vi "4024_Module_configure.vi"() -> ()   [LabVIEW 2020]
panel:
  in  "Output Range":u16(ring)=2 items=["30   0 to 20mA", "31   4 to 20mA", "32   0 to 10V"]
  in  "Ch Number":i8
  in  "Port Name":string="COM10"
  out "Reply":string
  out "ConfigStringSent":string
  in  "Address":u8
  # "This is a per channel configuration \nto be done after you have run \n4024_Module_INIT_configure.vi \n\nDon't run this vi when the ADAM 4024 is in the INIT mode"
  # "Happy reply starts \"!\"\nUnhappy reply starts \"?\""
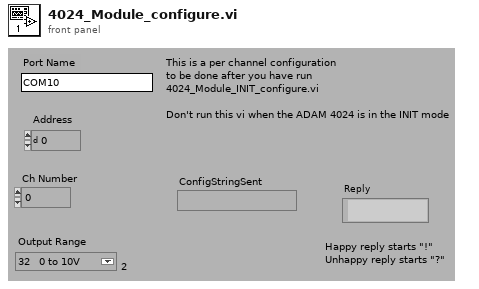
[diagram p1: front panel]
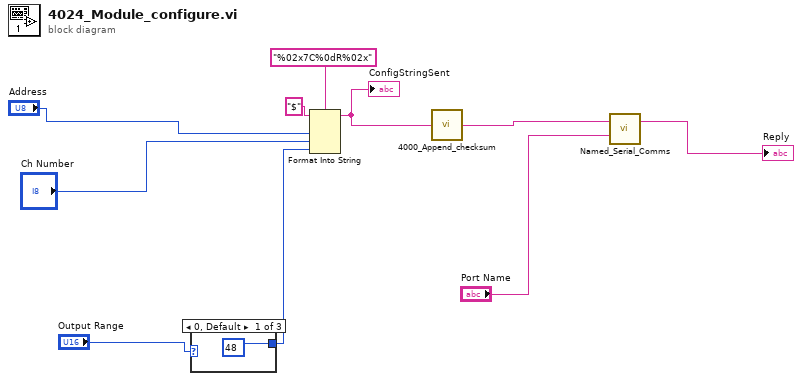
[diagram p0: block diagram]
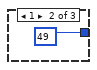
[diagram p2: hidden frame]
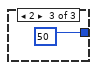
[diagram p3: hidden frame]
diagram:
  n1 = case shown="0, Default" "Output Range" {
    tunnel: [48 49 50] -> w1
    frame 0, Default {
    }
    frame 1 {
    }
    frame 2 {
    }
  }
  n2 = Format Into String(format string="%02x7C%0dR%02x", initial string="$", "Address", "Ch Number", w1) -> (resulting string=w8:string)  [unwired: 1 in, 1 out]
  "ConfigStringSent" <- w8
  n3 = call "4000_Append_checksum.vi"("ADAM command"=w8) -> ("ADAM string to send"=w6:string)
  n4 = call "Named_Serial_Comms.vi"("Write"=w6, "Port Name"="Port Name") -> ("Read"=→"Reply":string)  [unwired: 9 in, 4 out]
